vi "Configure Display Page.vi"(8 "error in":errorcluster, 10 "Display Page":u16(ring) items=["Measurement", "Measurement Setup", "BIN Measurement", "BIN Count", "BIN Setup", "LIST Measurement", "LIST Setup", "CORRECTION", "CATALOG", "ENLARGE", "System Config", "System Information"], 11 "VISA resource name":refnum<visa-resource-name>) -> (0 "error out":errorcluster, 3 "VISA resource name out":refnum<visa-resource-name>)   [LabVIEW 2021, in "LCR Meter.lvlib"]
doc: "Sets the Display Page."
uses:
  LCR Meter.lvlib
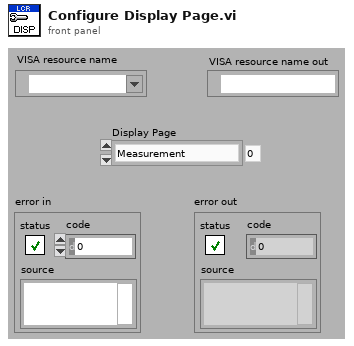
[diagram p1: front panel]
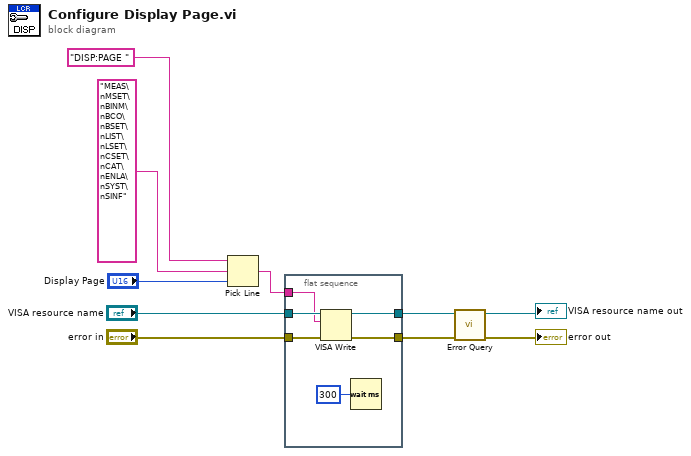
[diagram p0: block diagram]
diagram:
  n1 = Pick Line(string ("")="DISP:PAGE ", multi-line string="MEAS\nMSET\nBINM\nBCO\nBSET\nLIST\nLSET\nCSET\nCAT\nENLA\nSYST\nSINF", line index="Display Page") -> (output string=w3:string)
  n2 = flat-sequence {
    tunnel: "VISA resource name" -> [w16]
    tunnel: "error in" -> [w15]
    tunnel: [w13] -> w5
    tunnel: [w12] -> w4
    tunnel: w3 -> [w11]
    frame #0 {
      n3 = VISA Write(VISA resource name=w16, write buffer=w11, error in (no error)=w15) -> (VISA resource name out=w13:refnum<visa-resource-name>, error out=w12:errorcluster)  [unwired: 1 out]
      n4 = Wait (ms)(milliseconds to wait=u32 300) -> ()  [unwired: 1 out]
    }
  }
  n5 = call "Error Query.vi"("error in (no error)"=w4, "VISA resource name"=w5) -> ("error out"=→"error out":errorcluster, "VISA resource name out"=→"VISA resource name out":refnum<visa-resource-name>)  [unwired: 6 in, 2 out]
